vi "Write Level.vi"(8 "error in (no error)":errorcluster, 10 "Level":i32, 11 "Set O3 Level in":refnum<class "Set O3 Level.lvclass">) -> (0 "error out":errorcluster, 3 "Set O3 Level out":refnum<class "Set O3 Level.lvclass">)   [LabVIEW 2015, in "Set O3 Level.lvclass"]
uses:
  Set O3 Level.lvclass
  Set O3 Level.lvclass/Set O3 Level.ctl
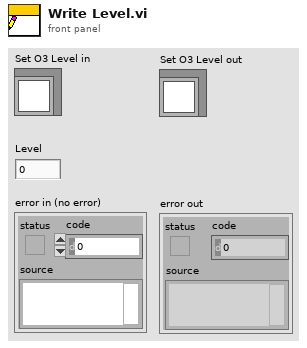
[diagram p1: front panel]
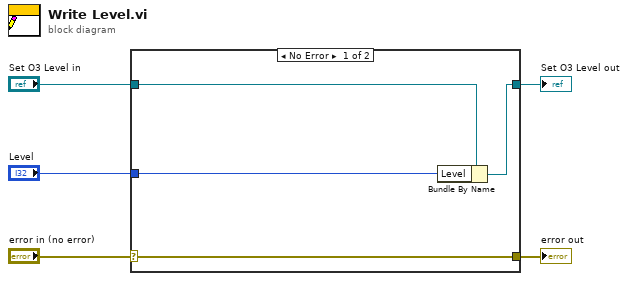
[diagram p0: block diagram]
diagram:
  n1 = case shown="No Error" "error in (no error)" {
    selector: "error in (no error)" -> [w9 w10]
    tunnel: [w9 w10] -> w4
    tunnel: [w7 w11] -> w2
    tunnel: "Set O3 Level in" -> [w8 w11]
    tunnel: "Level" -> [w6 _]
    frame No Error {
      n2 = Bundle By Name(cluster=w8, "Level"=w6) -> (w7:refnum<class "Set O3 Level.lvclass">)
    }
    frame Error {
    }
  }
  "error out" <- w4
  "Set O3 Level out" <- w2
